vi "Main.vi"(7 "sweep rate, /min":dbl=0.2, 8 "sweep to:":dbl=-0.5, 9 "sweep":T6(radio)=enum."time_sweep") -> ()   [LabVIEW 2017] (continued)
                n297 = property on="Hyper Channel" class="DigNum (strict)"("Value"=w243) -> ()  [unwired: 2 in, 2 out]
              }
            }
          }
          frame #3 {
            # "Update current value of measured channel"
            n298 = property on="Monitor" class="Bool (strict)"() -> ("Value"=w279:bool)  [unwired: 2 in, 2 out]
            n299 = case shown="True" w279 {
              frame False {
              }
              frame True {
                n300 = stacked-sequence {
                  frame #0 {
                    # "Prepare the display format"
                    n301 = local read "2636A smua meas v"() -> (w285:bool)
                    n302 = local read "2636A smub meas v"() -> (w283:bool)
                    n303 = local read "2636A smub meas i"() -> (w282:bool)
                    n304 = local read "2636A smua meas i"() -> (w284:bool)
                    n305 = property on="sweep" class="RadioBtnsControl (strict)"() -> ("Value"=w280:T6)  [unwired: 2 in, 2 out]
                    n306 = Compound Arithmetic op=OR(w285, w284, w283, w282) -> (w281:bool)
                    n307 = case shown="True" w281 {
                      frame False {
                      }
                      frame True {
                        # "opens session for 2636a system sourcemeter"
                        n308 = local read "2336A addr"() -> (w334:refnum<visa-resource-name>)
                        n309 = VISA Close(VISA resource name=w334) -> ()  [unwired: 1 in, 1 out]
                      }
                    }
                    n310 = case shown="\"iTC\"" w280 {
                      frame "2400_1" {
                        # "add label for the first column in the datafile"
                        n311 = stacked-sequence {
                          frame #0 {
                            n312 = property on="data_caption" class="Str"("Value"="") -> ()  [unwired: 2 in, 2 out]
                            n313 = property on="Figure_axis" class="Arr (strict)"("Value"=string[] [] ("Figure_axis_string")) -> ()  [unwired: 2 in, 2 out]
                          }
                          frame #1 {
                            w288 = "V_sweep_2400_1" ("V_sweep")
                            n314 = Concatenate Strings(w288, "\t") -> (w290:string)
                            n315 = Build Array(w288) -> (w289:string[])
                            n316 = property on="data_caption" class="Str"("Value"=w290) -> ()  [unwired: 2 in, 2 out]
                            n317 = property on="Figure_axis" class="Arr (strict)"("Value"=w289) -> ()  [unwired: 2 in, 2 out]
                          }
                        }
                      }
                      frame "2400_2" {
                        n318 = stacked-sequence {
                          frame #0 {
                            n319 = property on="data_caption" class="Str"("Value"="") -> ()  [unwired: 2 in, 2 out]
                            n320 = property on="Figure_axis" class="Arr (strict)"("Value"=string[] [] ("Figure_axis_string")) -> ()  [unwired: 2 in, 2 out]
                          }
                          frame #1 {
                            w294 = "V_sweep_2400_2" ("V_sweep")
                            n321 = Build Array(w294) -> (w295:string[])
                            n322 = Concatenate Strings(w294, "\t") -> (w297:string)
                            n323 = property on="Figure_axis" class="Arr (strict)"("Value"=w295) -> ()  [unwired: 2 in, 2 out]
                            n324 = property on="data_caption" class="Str"("Value"=w297) -> ()  [unwired: 2 in, 2 out]
                          }
                        }
                      }
                      frame "2400_3" {
                        n325 = stacked-sequence {
                          frame #0 {
                            n326 = property on="data_caption" class="Str"("Value"="") -> ()  [unwired: 2 in, 2 out]
                            n327 = property on="Figure_axis" class="Arr (strict)"("Value"=string[] [] ("Figure_axis_string")) -> ()  [unwired: 2 in, 2 out]
                          }
                          frame #1 {
                            w300 = "V_sweep_2400_3" ("V_sweep")
                            n328 = Concatenate Strings(w300, "\t") -> (w303:string)
                            n329 = Build Array(w300) -> (w301:string[])
                            n330 = property on="data_caption" class="Str"("Value"=w303) -> ()  [unwired: 2 in, 2 out]
                            n331 = property on="Figure_axis" class="Arr (strict)"("Value"=w301) -> ()  [unwired: 2 in, 2 out]
                          }
                        }
                      }
                      frame "2636a_smua" {
                        n332 = stacked-sequence {
                          frame #0 {
                            n333 = property on="data_caption" class="Str"("Value"="") -> ()  [unwired: 2 in, 2 out]
                            n334 = property on="Figure_axis" class="Arr (strict)"("Value"=string[] [] ("Figure_axis_string")) -> ()  [unwired: 2 in, 2 out]
                          }
                          frame #1 {
                            w306 = "V_sweep_2636a_smua" ("V_sweep")
                            n335 = Concatenate Strings(w306, "\t") -> (w309:string)
                            n336 = Build Array(w306) -> (w307:string[])
                            n337 = property on="data_caption" class="Str"("Value"=w309) -> ()  [unwired: 2 in, 2 out]
                            n338 = property on="Figure_axis" class="Arr (strict)"("Value"=w307) -> ()  [unwired: 2 in, 2 out]
                          }
                        }
                      }
                      frame "2636a_smub" {
                        n339 = stacked-sequence {
                          frame #0 {
                            n340 = property on="data_caption" class="Str"("Value"="") -> ()  [unwired: 2 in, 2 out]
                            n341 = property on="Figure_axis" class="Arr (strict)"("Value"=string[] [] ("Figure_axis_string")) -> ()  [unwired: 2 in, 2 out]
                          }
                          frame #1 {
                            w312 = "V_sweep_2636a_smub" ("V_sweep")
                            n342 = Build Array(w312) -> (w313:string[])
                            n343 = Concatenate Strings(w312, "\t") -> (w315:string)
                            n344 = property on="Figure_axis" class="Arr (strict)"("Value"=w313) -> ()  [unwired: 2 in, 2 out]
                            n345 = property on="data_caption" class="Str"("Value"=w315) -> ()  [unwired: 2 in, 2 out]
                          }
                        }
                      }
                      frame "time_sweep", Default {
                        n346 = stacked-sequence {
                          frame #0 {
                            n347 = property on="data_caption" class="Str"("Value"="") -> ()  [unwired: 2 in, 2 out]
                            n348 = property on="Figure_axis" class="Arr (strict)"("Value"=string[] [] ("Figure_axis_string")) -> ()  [unwired: 2 in, 2 out]
                          }
                          frame #1 {
                            w318 = "time_sweep" ("V_sweep")
                            n349 = Build Array(w318) -> (w319:string[])
                            n350 = Concatenate Strings(w318, "\t") -> (w320:string)
                            n351 = property on="Figure_axis" class="Arr (strict)"("Value"=w319) -> ()  [unwired: 2 in, 2 out]
                            n352 = property on="data_caption" class="Str"("Value"=w320) -> ()  [unwired: 2 in, 2 out]
                          }
                        }
                      }
                      frame "iPS" {
                        # "sweep iPS"
                        n353 = stacked-sequence {
                          frame #0 {
                            n354 = property on="data_caption" class="Str"("Value"="") -> ()  [unwired: 2 in, 2 out]
                            n355 = property on="Figure_axis" class="Arr (strict)"("Value"=string[] [] ("Figure_axis_string")) -> ()  [unwired: 2 in, 2 out]
                          }
                          frame #1 {
                            w324 = "iPS_OutputField" ("V_sweep")
                            n356 = Build Array(w324) -> (w325:string[])
                            n357 = Concatenate Strings(w324, "\t") -> (w327:string)
                            n358 = property on="Figure_axis" class="Arr (strict)"("Value"=w325) -> ()  [unwired: 2 in, 2 out]
                            n359 = property on="data_caption" class="Str"("Value"=w327) -> ()  [unwired: 2 in, 2 out]
                          }
                        }
                      }
                      frame "iTC" {
                        n360 = stacked-sequence {
                          frame #0 {
                            n361 = property on="data_caption" class="Str"("Value"="") -> ()  [unwired: 2 in, 2 out]
                            n362 = property on="Figure_axis" class="Arr (strict)"("Value"=string[] ["", "SR830_1_ip", "SR830_1_oop", "SR830_2_ip", "SR830_2_oop", "2461_meas_v", "2461_meas_i", "2636A_smua_v", "2636A_smua_i", "formula"] ("Figure_axis")) -> ()  [unwired: 2 in, 2 out]
                          }
                          frame #1 {
                            w332 = "iTC_sample"
                            n363 = Build Array(w332) -> (w331:string[])
                            n364 = Concatenate Strings(w332, "\t") -> (w330:string)
                            n365 = property on="data_caption" class="Str"("Value"=w330) -> ()  [unwired: 2 in, 2 out]
                            n366 = property on="Figure_axis" class="Arr (strict)"("Value"=w331) -> ()  [unwired: 2 in, 2 out]
                          }
                        }
                      }
                    }
                  }
                  frame #1 {
                    # "this part constructs the first (text) line for the data file with names of all measured variables,\nalso constructs a text array contaning names of all measured variable for the \"ring\" (so parameter can be selected and plotted)"
                    n367 = stacked-sequence {
                      tunnel: [w335 _ _ _ _ _ _ _ _ _ _ _ _ _ _ _ _ _ _ _ _ _ _ _ _ _ _ _ _ _ _ _ _ _ _ _ _ _ _ _ _ _ _ _ _ _ _ _ _ _ _ _] -> _
                      frame #0 {
                        # "SR830 1 in phase (SR830_1_ip)"
                        n368 = local read "SR830 1 ip"() -> (w340:bool)
                        n369 = property on="Figure_axis" class="Arr (strict)"() -> ("Value"=w337:string[])  [unwired: 2 in, 2 out]
                        n370 = property on="data_caption" class="Str"() -> ("Value"=w339:string)  [unwired: 2 in, 2 out]
                        n371 = case shown="True" w340 {
                          tunnel: w339 -> [w342 w348]
                          tunnel: [w342 w347] -> w338
                          tunnel: w337 -> [w341 w345]
                          tunnel: [w341 w343] -> w336
                          frame False {
                            # "not measure SR830 1 in phase signal (SR830_1_ip)"
                          }
                          frame True {
                            w344 = "SR830_1_ip"
                            # "measure SR830 1 in phase signal (SR830_1_ip)"
                            n372 = local read "SR830 1 addr"() -> (w349:u8)
                            n373 = Number To Decimal String(number=w349) -> (decimal integer string=w350:string)  [unwired: 1 in]
                            n374 = GPIB Clear(3:w350) -> ()  [unwired: 1 in, 2 out]
                            n375 = Build Array (concatenate)(w345, w344) -> (w343:string[])
                            n376 = Concatenate Strings(w348, w344, "\t") -> (w347:string)
                          }
                        }
                        n377 = property on="Figure_axis" class="Arr (strict)"("Value"=w336) -> ()  [unwired: 2 in, 2 out]
                        n378 = property on="data_caption" class="Str"("Value"=w338) -> (error out=w335:errorcluster)  [unwired: 2 in, 1 out]
                      }
                      frame #1 {
                        # "SR830 1 out of phase (SR830_1_oop)"
                        n379 = local read "SR830 1 oop"() -> (w355:bool)
                        n380 = property on="Figure_axis" class="Arr (strict)"() -> ("Value"=w352:string[])  [unwired: 2 in, 2 out]
                        n381 = property on="data_caption" class="Str"() -> ("Value"=w354:string)  [unwired: 2 in, 2 out]
                        n382 = case shown="False" w355 {
                          tunnel: w354 -> [w357 w363]
                          tunnel: [w357 w362] -> w353
                          tunnel: w352 -> [w356 w360]
                          tunnel: [w356 w358] -> w351
                          frame False {
                            # "not measure SR830 1 out of phase signal (SR830_1_oop)"
                          }
                          frame True {
                            w359 = "SR830_1_oop"
                            # "measure SR830 1 out of phase signal (SR830_1_oop)"
                            n383 = local read "SR830 1 addr"() -> (w364:u8)
                            n384 = Number To Decimal String(number=w364) -> (decimal integer string=w365:string)  [unwired: 1 in]
                            n385 = GPIB Clear(3:w365) -> ()  [unwired: 1 in, 2 out]
                            n386 = Build Array (concatenate)(w360, w359) -> (w358:string[])
                            n387 = Concatenate Strings(w363, w359, "\t") -> (w362:string)
                          }
                        }
                        n388 = property on="Figure_axis" class="Arr (strict)"("Value"=w351) -> ()  [unwired: 2 in, 2 out]
                        n389 = property on="data_caption" class="Str"("Value"=w353) -> ()  [unwired: 2 in, 2 out]
                      }
                      frame #2 {
                        # "SR830 2 in phase (SR830_2_ip)"
                        n390 = local read "SR830 2 ip"() -> (w370:bool)
                        n391 = property on="Figure_axis" class="Arr (strict)"() -> ("Value"=w367:string[])  [unwired: 2 in, 2 out]
                        n392 = property on="data_caption" class="Str"() -> ("Value"=w369:string)  [unwired: 2 in, 2 out]
                        n393 = case shown="True" w370 {
                          tunnel: w369 -> [w372 w378]
                          tunnel: [w372 w377] -> w368
                          tunnel: w367 -> [w371 w375]
                          tunnel: [w371 w373] -> w366
                          frame False {
                            # "not measure SR830 2 in phase signal (SR830_2_ip)"
                          }
                          frame True {
                            w374 = "SR830_2_ip"
                            # "measure SR830 2 in phase signal (SR830_2_ip)"
                            n394 = local read "SR830 2 addr"() -> (w379:u8)
                            n395 = Number To Decimal String(number=w379) -> (decimal integer string=w380:string)  [unwired: 1 in]
                            n396 = GPIB Clear(3:w380) -> ()  [unwired: 1 in, 2 out]
                            n397 = Build Array (concatenate)(w375, w374) -> (w373:string[])
                            n398 = Concatenate Strings(w378, w374, "\t") -> (w377:string)
                          }
                        }
                        n399 = property on="Figure_axis" class="Arr (strict)"("Value"=w366) -> ()  [unwired: 2 in, 2 out]
                        n400 = property on="data_caption" class="Str"("Value"=w368) -> ()  [unwired: 2 in, 2 out]
                      }
                      frame #3 {
                        # "SR830 2 out of phase (SR830_2_oop)"
                        n401 = local read "SR830 2 oop"() -> (w385:bool)
                        n402 = property on="Figure_axis" class="Arr (strict)"() -> ("Value"=w382:string[])  [unwired: 2 in, 2 out]
                        n403 = property on="data_caption" class="Str"() -> ("Value"=w384:string)  [unwired: 2 in, 2 out]
                        n404 = case shown="False" w385 {
                          tunnel: w384 -> [w387 w393]
                          tunnel: [w387 w392] -> w383
                          tunnel: w382 -> [w386 w390]
                          tunnel: [w386 w388] -> w381
                          frame False {
                            # "not measure SR830 2 out of phase signal (SR830_2_oop)"
                          }
                          frame True {
                            w389 = "SR830_2_oop"
                            # "measure SR830 2 out of phase signal (SR830_2_oop)"
                            n405 = local read "SR830 2 addr"() -> (w394:u8)
                            n406 = Number To Decimal String(number=w394) -> (decimal integer string=w395:string)  [unwired: 1 in]
                            n407 = GPIB Clear(3:w395) -> ()  [unwired: 1 in, 2 out]
                            n408 = Build Array (concatenate)(w390, w389) -> (w388:string[])
                            n409 = Concatenate Strings(w393, w389, "\t") -> (w392:string)
                          }
                        }
                        n410 = property on="Figure_axis" class="Arr (strict)"("Value"=w381) -> ()  [unwired: 2 in, 2 out]
                        n411 = property on="data_caption" class="Str"("Value"=w383) -> ()  [unwired: 2 in, 2 out]
                      }
                      frame #4 {
                        # "SR830 3 in phase (SR830_3_ip)"
                        n412 = local read "SR830 3 ip"() -> (w400:bool)
                        n413 = property on="Figure_axis" class="Arr (strict)"() -> ("Value"=w397:string[])  [unwired: 2 in, 2 out]
                        n414 = property on="data_caption" class="Str"() -> ("Value"=w399:string)  [unwired: 2 in, 2 out]
                        n415 = case shown="True" w400 {
                          tunnel: w399 -> [w402 w408]
                          tunnel: [w402 w407] -> w398
                          tunnel: w397 -> [w401 w405]
                          tunnel: [w401 w403] -> w396
                          frame False {
                            # "not measure SR830 3 in phase signal (SR830_3_ip)"
                          }
                          frame True {
                            w404 = "SR830_3_ip"
                            # "measure SR830 3 in phase signal (SR830_3_ip)"
                            n416 = local read "SR830 3 addr"() -> (w409:u8)
                            n417 = Number To Decimal String(number=w409) -> (decimal integer string=w410:string)  [unwired: 1 in]
                            n418 = GPIB Clear(3:w410) -> ()  [unwired: 1 in, 2 out]
                            n419 = Build Array (concatenate)(w405, w404) -> (w403:string[])
                            n420 = Concatenate Strings(w408, w404, "\t") -> (w407:string)
                          }
                        }
                        n421 = property on="Figure_axis" class="Arr (strict)"("Value"=w396) -> ()  [unwired: 2 in, 2 out]
                        n422 = property on="data_caption" class="Str"("Value"=w398) -> ()  [unwired: 2 in, 2 out]
                      }
                      frame #5 {
                        # "SR830 3 out of phase (SR830_3_oop)"
                        n423 = local read "SR830 3 oop"() -> (w415:bool)
                        n424 = property on="Figure_axis" class="Arr (strict)"() -> ("Value"=w412:string[])  [unwired: 2 in, 2 out]
                        n425 = property on="data_caption" class="Str"() -> ("Value"=w414:string)  [unwired: 2 in, 2 out]
                        n426 = case shown="True" w415 {
                          tunnel: w414 -> [w417 w423]
                          tunnel: [w417 w422] -> w413
                          tunnel: w412 -> [w416 w420]
                          tunnel: [w416 w418] -> w411
                          frame False {
                            # "not measure SR830 3 out of phase signal (SR830_3_oop)"
                          }
                          frame True {
                            w419 = "SR830_3_oop"
                            # "measure SR830 3 out phase signal (SR830_3_oop)"
                            n427 = local read "SR830 3 addr"() -> (w424:u8)
                            n428 = Number To Decimal String(number=w424) -> (decimal integer string=w425:string)  [unwired: 1 in]
                            n429 = GPIB Clear(3:w425) -> ()  [unwired: 1 in, 2 out]
                            n430 = Build Array (concatenate)(w420, w419) -> (w418:string[])
                            n431 = Concatenate Strings(w423, w419, "\t") -> (w422:string)
                          }
                        }
                        n432 = property on="Figure_axis" class="Arr (strict)"("Value"=w411) -> ()  [unwired: 2 in, 2 out]
                        n433 = property on="data_caption" class="Str"("Value"=w413) -> ()  [unwired: 2 in, 2 out]
                      }
                      frame #6 {
                        # "SR830 4 in phase (SR830_4_ip)"
                        n434 = local read "SR830 4 ip"() -> (w430:bool)
                        n435 = property on="Figure_axis" class="Arr (strict)"() -> ("Value"=w427:string[])  [unwired: 2 in, 2 out]
                        n436 = property on="data_caption" class="Str"() -> ("Value"=w429:string)  [unwired: 2 in, 2 out]
                        n437 = case shown="False" w430 {
                          tunnel: w429 -> [w432 w438]
                          tunnel: [w432 w437] -> w428
                          tunnel: w427 -> [w431 w435]
                          tunnel: [w431 w433] -> w426
                          frame False {
                            # "not measure SR830 4 in phase signal (SR830_4_ip)"
                          }
                          frame True {
                            w434 = "SR830_4_ip"
                            # "measure SR830 4 in phase signal (SR830_4_ip)"
                            n438 = local read "SR830 4 addr"() -> (w439:u8)
                            n439 = Number To Decimal String(number=w439) -> (decimal integer string=w440:string)  [unwired: 1 in]
                            n440 = GPIB Clear(3:w440) -> ()  [unwired: 1 in, 2 out]
                            n441 = Build Array (concatenate)(w435, w434) -> (w433:string[])
                            n442 = Concatenate Strings(w438, w434, "\t") -> (w437:string)
                          }
                        }
                        n443 = property on="Figure_axis" class="Arr (strict)"("Value"=w426) -> ()  [unwired: 2 in, 2 out]
                        n444 = property on="data_caption" class="Str"("Value"=w428) -> ()  [unwired: 2 in, 2 out]
                      }
                      frame #7 {
                        # "SR830 4 out of phase (SR830_4_oop)"
                        n445 = local read "SR830 4 oop"() -> (w445:bool)
                        n446 = property on="Figure_axis" class="Arr (strict)"() -> ("Value"=w442:string[])  [unwired: 2 in, 2 out]
                        n447 = property on="data_caption" class="Str"() -> ("Value"=w444:string)  [unwired: 2 in, 2 out]
                        n448 = case shown="False" w445 {
                          tunnel: w444 -> [w447 w453]
                          tunnel: [w447 w452] -> w443
                          tunnel: w442 -> [w446 w450]
                          tunnel: [w446 w448] -> w441
                          frame False {
                            # "not measure SR830 4 out of phase signal (SR830_4_oop)"
                          }
                          frame True {
                            w449 = "SR830_4_oop"
                            # "measure SR830 4 out of phase signal (SR830_4_oop)"
                            n449 = local read "SR830 4 addr"() -> (w454:u8)
                            n450 = Number To Decimal String(number=w454) -> (decimal integer string=w455:string)  [unwired: 1 in]
                            n451 = GPIB Clear(3:w455) -> ()  [unwired: 1 in, 2 out]
                            n452 = Build Array (concatenate)(w450, w449) -> (w448:string[])
                            n453 = Concatenate Strings(w453, w449, "\t") -> (w452:string)
                          }
                        }
                        n454 = property on="Figure_axis" class="Arr (strict)"("Value"=w441) -> ()  [unwired: 2 in, 2 out]
                        n455 = property on="data_caption" class="Str"("Value"=w443) -> ()  [unwired: 2 in, 2 out]
                      }
                      frame #8 {
                        # "SR830 5 in phase (SR830_5_ip)"
                        n456 = local read "SR830 5 ip"() -> (w460:bool)
                        n457 = property on="Figure_axis" class="Arr (strict)"() -> ("Value"=w457:string[])  [unwired: 2 in, 2 out]
                        n458 = property on="data_caption" class="Str"() -> ("Value"=w459:string)  [unwired: 2 in, 2 out]
                        n459 = case shown="True" w460 {
                          tunnel: w459 -> [w462 w468]
                          tunnel: [w462 w467] -> w458
                          tunnel: w457 -> [w461 w465]
                          tunnel: [w461 w463] -> w456
                          frame False {
                            # "not measure SR830 5 in phase signal (SR830_5_ip)"
                          }
                          frame True {
                            w464 = "SR830_5_ip"
                            # "measure SR830 5 in phase signal (SR830_5_ip)"
                            n460 = local read "SR830 5 addr"() -> (w469:u8)
                            n461 = Number To Decimal String(number=w469) -> (decimal integer string=w470:string)  [unwired: 1 in]
                            n462 = GPIB Clear(3:w470) -> ()  [unwired: 1 in, 2 out]
                            n463 = Build Array (concatenate)(w465, w464) -> (w463:string[])
                            n464 = Concatenate Strings(w468, w464, "\t") -> (w467:string)
                          }
                        }
                        n465 = property on="Figure_axis" class="Arr (strict)"("Value"=w456) -> ()  [unwired: 2 in, 2 out]
                        n466 = property on="data_caption" class="Str"("Value"=w458) -> ()  [unwired: 2 in, 2 out]
                      }
                      frame #9 {
                        # "SR830 5 out of phase (SR830_5_oop)"
                        n467 = local read "SR830 5 oop"() -> (w475:bool)
                        n468 = property on="Figure_axis" class="Arr (strict)"() -> ("Value"=w472:string[])  [unwired: 2 in, 2 out]
                        n469 = property on="data_caption" class="Str"() -> ("Value"=w474:string)  [unwired: 2 in, 2 out]
                        n470 = case shown="True" w475 {
                          tunnel: w474 -> [w477 w483]
                          tunnel: [w477 w482] -> w473
                          tunnel: w472 -> [w476 w480]
                          tunnel: [w476 w478] -> w471
                          frame False {
                            # "not measure SR830 5 out of phase signal (SR830_5_oop)"
                          }
                          frame True {
                            w479 = "SR830_5_oop"
                            # "measure SR830 5 out of phase signal (SR830_5_oop)"
                            n471 = local read "SR830 5 addr"() -> (w484:u8)
                            n472 = Number To Decimal String(number=w484) -> (decimal integer string=w485:string)  [unwired: 1 in]
                            n473 = GPIB Clear(3:w485) -> ()  [unwired: 1 in, 2 out]
                            n474 = Build Array (concatenate)(w480, w479) -> (w478:string[])
                            n475 = Concatenate Strings(w483, w479, "\t") -> (w482:string)
                          }
                        }
                        n476 = property on="Figure_axis" class="Arr (strict)"("Value"=w471) -> ()  [unwired: 2 in, 2 out]
                        n477 = property on="data_caption" class="Str"("Value"=w473) -> ()  [unwired: 2 in, 2 out]
                      }
                      frame #10 {
                        # "SR830 6 in phase (SR830_6_ip)"
                        n478 = property on="SR830_6_ip" class="Bool (strict)"() -> ("Value"=w486:bool)  [unwired: 2 in, 2 out]
                        n479 = property on="Figure_axis" class="Arr (strict)"() -> ("Value"=w488:string[])  [unwired: 2 in, 2 out]
                        n480 = property on="data_caption" class="Str"() -> ("Value"=w490:string)  [unwired: 2 in, 2 out]
                        n481 = case shown="True" w486 {
                          tunnel: w490 -> [w492 w498]
                          tunnel: [w492 w497] -> w489
                          tunnel: w488 -> [w491 w495]
                          tunnel: [w491 w493] -> w487
                          frame False {
                            # "not measure SR830 6 in phase signal (SR830_6_ip)"
                          }
                          frame True {
                            w494 = "SR830_6_ip"
                            # "measure SR830 6 in phase signal (SR830_6_ip)"
                            n482 = local read "SR830_6"() -> (w499:u8)
                            n483 = Number To Decimal String(number=w499) -> (decimal integer string=w500:string)  [unwired: 1 in]
                            n484 = GPIB Clear(3:w500) -> ()  [unwired: 1 in, 2 out]
                            n485 = Build Array (concatenate)(w495, w494) -> (w493:string[])
                            n486 = Concatenate Strings(w498, w494, "\t") -> (w497:string)
                          }
                        }
                        n487 = property on="Figure_axis" class="Arr (strict)"("Value"=w487) -> ()  [unwired: 2 in, 2 out]
                        n488 = property on="data_caption" class="Str"("Value"=w489) -> ()  [unwired: 2 in, 2 out]
                      }
                      frame #11 {
                        # "SR830 6 out of phase (SR830_6_oop)"
                        n489 = local read "SR830_6_oop"() -> (w505:bool)
                        n490 = property on="Figure_axis" class="Arr (strict)"() -> ("Value"=w502:string[])  [unwired: 2 in, 2 out]
                        n491 = property on="data_caption" class="Str"() -> ("Value"=w504:string)  [unwired: 2 in, 2 out]
                        n492 = case shown="False" w505 {
                          tunnel: w504 -> [w507 w513]
                          tunnel: [w507 w512] -> w503
                          tunnel: w502 -> [w506 w510]
                          tunnel: [w506 w508] -> w501
                          frame False {
                            # "not measure SR830 6 out of phase signal (SR830_6_oop)"
                          }
                          frame True {
                            w509 = "SR830_6_oop"
                            # "measure SR830 6 out of phase signal (SR830_6_oop)"
                            n493 = local read "SR830_6"() -> (w514:u8)
                            n494 = Number To Decimal String(number=w514) -> (decimal integer string=w515:string)  [unwired: 1 in]
                            n495 = GPIB Clear(3:w515) -> ()  [unwired: 1 in, 2 out]
                            n496 = Build Array (concatenate)(w510, w509) -> (w508:string[])
                            n497 = Concatenate Strings(w513, w509, "\t") -> (w512:string)
                          }
                        }
                        n498 = property on="Figure_axis" class="Arr (strict)"("Value"=w501) -> ()  [unwired: 2 in, 2 out]
                        n499 = property on="data_caption" class="Str"("Value"=w503) -> ()  [unwired: 2 in, 2 out]
                      }
                      frame #12 {
                        # "SR830 7 in phase (SR830_7_ip)"
                        n500 = local read "SR830_7_ip"() -> (w516:bool)
                        n501 = property on="Figure_axis" class="Arr (strict)"() -> ("Value"=w518:string[])  [unwired: 2 in, 2 out]
                        n502 = property on="data_caption" class="Str"() -> ("Value"=w520:string)  [unwired: 2 in, 2 out]
                        n503 = case shown="True" w516 {
                          tunnel: w520 -> [w522 w528]
                          tunnel: [w522 w527] -> w519
                          tunnel: w518 -> [w521 w525]
                          tunnel: [w521 w523] -> w517
                          frame False {
                            # "not measure SR830 7 in phase signal (SR830_7_ip)"
                          }
                          frame True {
                            w524 = "SR830_7_ip"
                            # "measure SR830 7 in phase signal (SR830_7_ip)"
                            n504 = local read "SR830_7"() -> (w529:u8)
                            n505 = Number To Decimal String(number=w529) -> (decimal integer string=w530:string)  [unwired: 1 in]
                            n506 = GPIB Clear(3:w530) -> ()  [unwired: 1 in, 2 out]
                            n507 = Build Array (concatenate)(w525, w524) -> (w523:string[])
                            n508 = Concatenate Strings(w528, w524, "\t") -> (w527:string)
                          }
                        }
                        n509 = property on="Figure_axis" class="Arr (strict)"("Value"=w517) -> ()  [unwired: 2 in, 2 out]
                        n510 = property on="data_caption" class="Str"("Value"=w519) -> ()  [unwired: 2 in, 2 out]
                      }
                      frame #13 {
                        # "SR830 7 out of phase (SR830_7_oop)"
                        n511 = local read "SR830_7_oop"() -> (w535:bool)
                        n512 = property on="Figure_axis" class="Arr (strict)"() -> ("Value"=w532:string[])  [unwired: 2 in, 2 out]
                        n513 = property on="data_caption" class="Str"() -> ("Value"=w534:string)  [unwired: 2 in, 2 out]
                        n514 = case shown="True" w535 {
                          tunnel: w534 -> [w537 w543]
                          tunnel: [w537 w542] -> w533
                          tunnel: w532 -> [w536 w540]
                          tunnel: [w536 w538] -> w531
                          frame False {
                            # "not measure SR830 7 out of phase signal (SR830_7_oop)"
                          }
                          frame True {
                            w539 = "SR830_7_oop"
                            # "measure SR830 7 out of phase signal (SR830_7_oop)"
                            n515 = local read "SR830_7"() -> (w544:u8)
                            n516 = Number To Decimal String(number=w544) -> (decimal integer string=w545:string)  [unwired: 1 in]
                            n517 = GPIB Clear(3:w545) -> ()  [unwired: 1 in, 2 out]
                            n518 = Build Array (concatenate)(w540, w539) -> (w538:string[])
                            n519 = Concatenate Strings(w543, w539, "\t") -> (w542:string)
                          }
                        }
                        n520 = property on="Figure_axis" class="Arr (strict)"("Value"=w531) -> ()  [unwired: 2 in, 2 out]
                        n521 = property on="data_caption" class="Str"("Value"=w533) -> ()  [unwired: 2 in, 2 out]
                      }
                      frame #14 {
                        # "SR830 8 in phase (SR830_8_ip)"
                        n522 = local read "SR830_8_ip"() -> (w546:bool)
                        n523 = property on="Figure_axis" class="Arr (strict)"() -> ("Value"=w548:string[])  [unwired: 2 in, 2 out]
                        n524 = property on="data_caption" class="Str"() -> ("Value"=w550:string)  [unwired: 2 in, 2 out]
                        n525 = case shown="True" w546 {
                          tunnel: w550 -> [w552 w558]
                          tunnel: [w552 w557] -> w549
                          tunnel: w548 -> [w551 w555]
                          tunnel: [w551 w553] -> w547
                          frame False {
                            # "not measure SR830 8 in phase signal (SR830_8_ip)"
                          }
                          frame True {
                            w554 = "SR830_8_ip"
                            # "measure SR830 8 in phase signal (SR830_8_ip)"
                            n526 = local read "SR830_8"() -> (w559:u8)
                            n527 = Number To Decimal String(number=w559) -> (decimal integer string=w560:string)  [unwired: 1 in]
                            n528 = GPIB Clear(3:w560) -> ()  [unwired: 1 in, 2 out]
                            n529 = Build Array (concatenate)(w555, w554) -> (w553:string[])
                            n530 = Concatenate Strings(w558, w554, "\t") -> (w557:string)
                          }
                        }
                        n531 = property on="Figure_axis" class="Arr (strict)"("Value"=w547) -> ()  [unwired: 2 in, 2 out]
                        n532 = property on="data_caption" class="Str"("Value"=w549) -> ()  [unwired: 2 in, 2 out]
                      }
                      frame #15 {
                        # "SR830 8 out phase (SR830_8_oop)"
                        n533 = local read "SR830_8_oop"() -> (w561:bool)
                        n534 = property on="Figure_axis" class="Arr (strict)"() -> ("Value"=w563:string[])  [unwired: 2 in, 2 out]
                        n535 = property on="data_caption" class="Str"() -> ("Value"=w565:string)  [unwired: 2 in, 2 out]
                        n536 = case shown="True" w561 {
                          tunnel: w565 -> [w567 w573]
                          tunnel: [w567 w572] -> w564
                          tunnel: w563 -> [w566 w570]
                          tunnel: [w566 w568] -> w562
                          frame False {
                            # "not measure SR830 8 out phase signal (SR830_8_oop)"
                          }
                          frame True {
                            w569 = "SR830_8_oop"
                            # "measure SR830 8 out phase signal (SR830_8_00p)"
                            n537 = local read "SR830_8"() -> (w574:u8)
                            n538 = Number To Decimal String(number=w574) -> (decimal integer string=w575:string)  [unwired: 1 in]
                            n539 = GPIB Clear(3:w575) -> ()  [unwired: 1 in, 2 out]
                            n540 = Build Array (concatenate)(w570, w569) -> (w568:string[])
                            n541 = Concatenate Strings(w573, w569, "\t") -> (w572:string)
                          }
                        }
                        n542 = property on="Figure_axis" class="Arr (strict)"("Value"=w562) -> ()  [unwired: 2 in, 2 out]
                        n543 = property on="data_caption" class="Str"("Value"=w564) -> ()  [unwired: 2 in, 2 out]
                      }
                      frame #16 {
                        # "MFLI_V1"
                        n544 = property on="MFLI_1" class="Str" props=["Value"]() -> ()  [unwired: 2 in, 3 out]
                        n545 = property on="MFLI_V1" class="Bool (strict)"() -> ("Value"=w576:bool)  [unwired: 2 in, 2 out]
                        n546 = property on="data_caption" class="Str"() -> ("Value"=w580:string)  [unwired: 2 in, 2 out]
                        n547 = property on="Figure_axis" class="Arr (strict)"() -> ("Value"=w578:string[])  [unwired: 2 in, 2 out]
                        n548 = case shown="True" w576 {
                          tunnel: w580 -> [w582 w592]
                          tunnel: [w582 w591] -> w579
                          tunnel: w578 -> [w581 w590]
                          tunnel: [w581 w589] -> w577
                          frame False {
                            # "not measure 2461 voltage (2461_meas_v)"
                          }
                          frame True {
                            w587 = "MFLI_Vy_1"
                            w588 = "MFLI_Vx_1"
                            w586 = "\t"
                            w585 = "MFLI_freq_1"
                            n549 = property on="HandleOut" class="Clust (strict)"() -> ("Value"=w584:T5)  [unwired: 2 in, 2 out]
                            n550 = Unbundle(w584) -> ("Connected"=w583:bool)  [unwired: 5 out]
                            n551 = case shown="False" w583 {
                              frame False {
                                n552 = property on="MFLI_1" class="Str"() -> ("Value"=w595:string)  [unwired: 2 in, 2 out]
                                n553 = call <instrlib>:"ziOpen.vi"("Address"=w595) -> ("HandleOut"=w594:T5)  [unwired: 3 in, 2 out]
                                n554 = call <instrlib>:"ziCheckVersion.vi"("Handle In"=w594) -> ("Handle Out"=w593:T5)  [unwired: 12 in, 2 out]
                                n555 = property on="HandleOut" class="Clust (strict)"("Value"=w593) -> ()  [unwired: 2 in, 2 out]
                              }
                              frame True {
                              }
                            }
                            n556 = Build Array (concatenate)(w590, w588, w587, w585) -> (w589:string[])
                            n557 = Concatenate Strings(w592, w588, w586, w587, w586, w585, w586) -> (w591:string)
                          }
                        }
                        n558 = property on="Figure_axis" class="Arr (strict)"("Value"=w577) -> ()  [unwired: 2 in, 2 out]
                        n559 = property on="data_caption" class="Str"("Value"=w579) -> ()  [unwired: 2 in, 2 out]
                      }
                      frame #17 {
                        # "MFLI_I1"
                        n560 = property on="MFLI_I1" class="Bool (strict)"() -> ("Value"=w596:bool)  [unwired: 2 in, 2 out]
                        n561 = property on="data_caption" class="Str"() -> ("Value"=w600:string)  [unwired: 2 in, 2 out]
                        n562 = property on="Figure_axis" class="Arr (strict)"() -> ("Value"=w598:string[])  [unwired: 2 in, 2 out]
                        n563 = case shown="True" w596 {
                          tunnel: w600 -> [w602 w612]
                          tunnel: [w602 w611] -> w599
                          tunnel: w598 -> [w601 w610]
                          tunnel: [w601 w609] -> w597
                          frame False {
                            # "not measure 2461 voltage (2461_meas_v)"
                          }
                          frame True {
                            w607 = "MFLI_Iy-1"
                            w608 = "MFLI_Ix_1"
                            w606 = "\t"
                            w605 = "MFLI_freq_1"
                            n564 = property on="HandleOut" class="Clust (strict)"() -> ("Value"=w604:T5)  [unwired: 2 in, 2 out]
                            n565 = Unbundle(w604) -> ("Connected"=w603:bool)  [unwired: 5 out]
                            n566 = case shown="False" w603 {
                              frame False {
                                n567 = property on="MFLI_1" class="Str"() -> ("Value"=w615:string)  [unwired: 2 in, 2 out]
                                n568 = call <instrlib>:"ziOpen.vi"("Address"=w615) -> ("HandleOut"=w614:T5)  [unwired: 3 in, 2 out]
                                n569 = call <instrlib>:"ziCheckVersion.vi"("Handle In"=w614) -> ("Handle Out"=w613:T5)  [unwired: 12 in, 2 out]
                                n570 = property on="HandleOut" class="Clust (strict)"("Value"=w613) -> ()  [unwired: 2 in, 2 out]
                              }
                              frame True {
                              }
                            }
                            n571 = Build Array (concatenate)(w610, w608, w607, w605) -> (w609:string[])
                            n572 = Concatenate Strings(w612, w608, w606, w607, w606, w605, w606) -> (w611:string)
                          }
                        }
                        n573 = property on="Figure_axis" class="Arr (strict)"("Value"=w597) -> ()  [unwired: 2 in, 2 out]
                        n574 = property on="data_caption" class="Str"("Value"=w599) -> ()  [unwired: 2 in, 2 out]
                      }
                      frame #18 {
                        # "MFLI_V 2"
                        n575 = local read "MFLI_V2"() -> (w616:bool)
                        n576 = property on="data_caption" class="Str"() -> ("Value"=w620:string)  [unwired: 2 in, 2 out]
                        n577 = property on="Figure_axis" class="Arr (strict)"() -> ("Value"=w618:string[])  [unwired: 2 in, 2 out]
                        n578 = case shown="True" w616 {
                          tunnel: w620 -> [w622 w632]
                          tunnel: [w622 w631] -> w619
                          tunnel: w618 -> [w621 w630]
                          tunnel: [w621 w629] -> w617
                          frame False {
                          }
                          frame True {
                            w627 = "MFLI_Vy_2"
                            w628 = "MFLI_Vx_2"
                            w626 = "\t"
                            w625 = "MFLI_freq_2"
                            n579 = property on="Handle Out 2" class="Clust (strict)"() -> ("Value"=w624:T5)  [unwired: 2 in, 2 out]
                            n580 = Unbundle(w624) -> ("Connected"=w623:bool)  [unwired: 5 out]
                            n581 = case shown="False" w623 {
                              frame False {
                                n582 = local read "MFLI_2"() -> (w633:string)
                                n583 = call <instrlib>:"ziOpen.vi"("Address"=w633) -> ("HandleOut"=w635:T5)  [unwired: 3 in, 2 out]
                                n584 = call <instrlib>:"ziCheckVersion.vi"("Handle In"=w635) -> ("Handle Out"=w634:T5)  [unwired: 12 in, 2 out]
                                n585 = property on="Handle Out 2" class="Clust (strict)"("Value"=w634) -> ()  [unwired: 2 in, 2 out]
                              }
                              frame True {
                              }
                            }
                            n586 = Build Array (concatenate)(w630, w628, w627, w625) -> (w629:string[])
                            n587 = Concatenate Strings(w632, w628, w626, w627, w626, w625, w626) -> (w631:string)
                          }
                        }
                        n588 = property on="Figure_axis" class="Arr (strict)"("Value"=w617) -> ()  [unwired: 2 in, 2 out]
                        n589 = property on="data_caption" class="Str"("Value"=w619) -> ()  [unwired: 2 in, 2 out]
                      }
                      frame #19 {
                        # "MFLI_I 2"
                        n590 = local read "MFLI_I2"() -> (w636:bool)
                        n591 = property on="data_caption" class="Str"() -> ("Value"=w640:string)  [unwired: 2 in, 2 out]
                        n592 = property on="Figure_axis" class="Arr (strict)"() -> ("Value"=w638:string[])  [unwired: 2 in, 2 out]
                        n593 = case shown="True" w636 {
                          tunnel: w640 -> [w642 w652]
                          tunnel: [w642 w651] -> w639
                          tunnel: w638 -> [w641 w650]
                          tunnel: [w641 w649] -> w637
                          frame False {
                            # "not measure 2461 voltage (2461_meas_v)"
                          }
                          frame True {
                            w647 = "MFLI_Iy_2"
                            w648 = "MFLI_Ix_2"
                            w646 = "\t"
                            w645 = "MFLI_freq_2"
                            n594 = property on="Handle Out 2" class="Clust (strict)"() -> ("Value"=w644:T5)  [unwired: 2 in, 2 out]
                            n595 = Unbundle(w644) -> ("Connected"=w643:bool)  [unwired: 5 out]
                            n596 = case shown="False" w643 {
                              frame False {
                                n597 = local read "MFLI_2"() -> (w653:string)
                                n598 = call <instrlib>:"ziOpen.vi"("Address"=w653) -> ("HandleOut"=w655:T5)  [unwired: 3 in, 2 out]
                                n599 = call <instrlib>:"ziCheckVersion.vi"("Handle In"=w655) -> ("Handle Out"=w654:T5)  [unwired: 12 in, 2 out]
                                n600 = property on="Handle Out 2" class="Clust (strict)"("Value"=w654) -> ()  [unwired: 2 in, 2 out]
                              }
                              frame True {
                              }
                            }
                            n601 = Build Array (concatenate)(w650, w648, w647, w645) -> (w649:string[])
                            n602 = Concatenate Strings(w652, w648, w646, w647, w646, w645, w646) -> (w651:string)
                          }
                        }
                        n603 = property on="Figure_axis" class="Arr (strict)"("Value"=w637) -> ()  [unwired: 2 in, 2 out]
                        n604 = property on="data_caption" class="Str"("Value"=w639) -> ()  [unwired: 2 in, 2 out]
                      }
                      frame #20 {
                        # "2400 1 voltage measure (2400_1_v)"
                        n605 = local read "2400 1 meas v"() -> (w660:bool)
                        n606 = property on="Figure_axis" class="Arr (strict)"() -> ("Value"=w657:string[])  [unwired: 2 in, 2 out]
                        n607 = property on="data_caption" class="Str"() -> ("Value"=w659:string)  [unwired: 2 in, 2 out]
                        n608 = case shown="False" w660 {
                          tunnel: w659 -> [w662 w668]
                          tunnel: [w662 w667] -> w658
                          tunnel: w657 -> [w661 w665]
                          tunnel: [w661 w663] -> w656
                          frame False {
                            # "not measure 2400 1 voltage (2400_1_v)"
                          }
                          frame True {
                            w664 = "2400_1_v"
                            # "measure 2400 1 voltage (2400_1_v)"
                            n609 = local read "2400 1 addr"() -> (w669:u8)
                            n610 = Number To Decimal String(number=w669) -> (decimal integer string=w670:string)  [unwired: 1 in]
                            n611 = GPIB Clear(3:w670) -> ()  [unwired: 1 in, 2 out]
                            n612 = Build Array (concatenate)(w665, w664) -> (w663:string[])
                            n613 = Concatenate Strings(w668, w664, "\t") -> (w667:string)
                          }
                        }
                        n614 = property on="Figure_axis" class="Arr (strict)"("Value"=w656) -> ()  [unwired: 2 in, 2 out]
                        n615 = property on="data_caption" class="Str"("Value"=w658) -> ()  [unwired: 2 in, 2 out]
                      }
                      frame #21 {
                        # "2400 1 current measure (2400_1_i)"
                        n616 = local read "2400 1 meas i"() -> (w675:bool)
                        n617 = property on="Figure_axis" class="Arr (strict)"() -> ("Value"=w672:string[])  [unwired: 2 in, 2 out]
                        n618 = property on="data_caption" class="Str"() -> ("Value"=w674:string)  [unwired: 2 in, 2 out]
                        n619 = case shown="False" w675 {
                          tunnel: w674 -> [w677 w683]
                          tunnel: [w677 w682] -> w673
                          tunnel: w672 -> [w676 w680]
                          tunnel: [w676 w678] -> w671
                          frame False {
                            # "not measure 2400 1 current (2400_1_i)"
                          }
                          frame True {
                            w679 = "2400_1_i"
                            # "measure 2400 1 current (2400_1_i)"
                            n620 = local read "2400 1 addr"() -> (w684:u8)
                            n621 = Number To Decimal String(number=w684) -> (decimal integer string=w685:string)  [unwired: 1 in]
                            n622 = GPIB Clear(3:w685) -> ()  [unwired: 1 in, 2 out]
                            n623 = Build Array (concatenate)(w680, w679) -> (w678:string[])
                            n624 = Concatenate Strings(w683, w679, "\t") -> (w682:string)
                          }
                        }
                        n625 = property on="Figure_axis" class="Arr (strict)"("Value"=w671) -> ()  [unwired: 2 in, 2 out]
                        n626 = property on="data_caption" class="Str"("Value"=w673) -> ()  [unwired: 2 in, 2 out]
                      }
                      frame #22 {
                        # "2400 2 voltage measure (2400_2_v)"
                        n627 = local read "2400 2 meas v"() -> (w690:bool)
                        n628 = property on="Figure_axis" class="Arr (strict)"() -> ("Value"=w687:string[])  [unwired: 2 in, 2 out]
                        n629 = property on="data_caption" class="Str"() -> ("Value"=w689:string)  [unwired: 2 in, 2 out]
                        n630 = case shown="False" w690 {
                          tunnel: w689 -> [w692 w698]
                          tunnel: [w692 w697] -> w688
                          tunnel: w687 -> [w691 w695]
                          tunnel: [w691 w693] -> w686
                          frame False {
                            # "not measure 2400 2 voltage (2400_2_v)"
                          }
                          frame True {
                            w694 = "2400_2_v"
                            # "measure 2400 2 voltage (2400_2_v)"
                            n631 = local read "2400 2 addr"() -> (w699:u8)
                            n632 = Number To Decimal String(number=w699) -> (decimal integer string=w700:string)  [unwired: 1 in]
                            n633 = GPIB Clear(3:w700) -> ()  [unwired: 1 in, 2 out]
                            n634 = Build Array (concatenate)(w695, w694) -> (w693:string[])
                            n635 = Concatenate Strings(w698, w694, "\t") -> (w697:string)
                          }
                        }
                        n636 = property on="Figure_axis" class="Arr (strict)"("Value"=w686) -> ()  [unwired: 2 in, 2 out]
                        n637 = property on="data_caption" class="Str"("Value"=w688) -> ()  [unwired: 2 in, 2 out]
                      }
                      frame #23 {
                        # "2400 2 current measure (2400_2_i)"
                        n638 = local read "2400 2 meas i"() -> (w705:bool)
                        n639 = property on="Figure_axis" class="Arr (strict)"() -> ("Value"=w702:string[])  [unwired: 2 in, 2 out]
                        n640 = property on="data_caption" class="Str"() -> ("Value"=w704:string)  [unwired: 2 in, 2 out]
                        n641 = case shown="False" w705 {
                          tunnel: w704 -> [w707 w713]
                          tunnel: [w707 w712] -> w703
                          tunnel: w702 -> [w706 w710]
                          tunnel: [w706 w708] -> w701
                          frame False {
                            # "not measure 2400 2 current (2400_2_i)"
                          }
                          frame True {
                            w709 = "2400_2_i"
                            # "measure 2400 2 current (2400_2_i)"
                            n642 = local read "2400 2 addr"() -> (w714:u8)
                            n643 = Number To Decimal String(number=w714) -> (decimal integer string=w715:string)  [unwired: 1 in]
                            n644 = GPIB Clear(3:w715) -> ()  [unwired: 1 in, 2 out]
                            n645 = Build Array (concatenate)(w710, w709) -> (w708:string[])
                            n646 = Concatenate Strings(w713, w709, "\t") -> (w712:string)
                          }
                        }
                        n647 = property on="Figure_axis" class="Arr (strict)"("Value"=w701) -> ()  [unwired: 2 in, 2 out]
                        n648 = property on="data_caption" class="Str"("Value"=w703) -> ()  [unwired: 2 in, 2 out]
                      }
                      frame #24 {
                        # "2400 3 voltage measure (2400_3_v)"
                        n649 = local read "2400 3 meas v"() -> (w720:bool)
                        n650 = property on="Figure_axis" class="Arr (strict)"() -> ("Value"=w717:string[])  [unwired: 2 in, 2 out]
                        n651 = property on="data_caption" class="Str"() -> ("Value"=w719:string)  [unwired: 2 in, 2 out]
                        n652 = case shown="False" w720 {
                          tunnel: w719 -> [w722 w728]
                          tunnel: [w722 w727] -> w718
                          tunnel: w717 -> [w721 w725]
                          tunnel: [w721 w723] -> w716
                          frame False {
                            # "not measure 2400 3 voltage (2400_3_v)"
                          }
                          frame True {
                            w724 = "2400_3_v"
                            # "measure 2400 3 voltage (2400_3_v)"
                            n653 = local read "2400 3 addr"() -> (w729:u8)
                            n654 = Number To Decimal String(number=w729) -> (decimal integer string=w730:string)  [unwired: 1 in]
                            n655 = GPIB Clear(3:w730) -> ()  [unwired: 1 in, 2 out]
                            n656 = Build Array (concatenate)(w725, w724) -> (w723:string[])
                            n657 = Concatenate Strings(w728, w724, "\t") -> (w727:string)
                          }
                        }
                        n658 = property on="Figure_axis" class="Arr (strict)"("Value"=w716) -> ()  [unwired: 2 in, 2 out]
                        n659 = property on="data_caption" class="Str"("Value"=w718) -> ()  [unwired: 2 in, 2 out]
                      }
                      frame #25 {
                        # "2400 3 current measure (2400_3_i)"
                        n660 = local read "2400 3 meas i"() -> (w735:bool)
                        n661 = property on="Figure_axis" class="Arr (strict)"() -> ("Value"=w732:string[])  [unwired: 2 in, 2 out]
                        n662 = property on="data_caption" class="Str"() -> ("Value"=w734:string)  [unwired: 2 in, 2 out]
                        n663 = case shown="True" w735 {
                          tunnel: w734 -> [w737 w743]
                          tunnel: [w737 w742] -> w733
                          tunnel: w732 -> [w736 w740]
                          tunnel: [w736 w738] -> w731
                          frame False {
                            # "not measure 2400 3 current (2400_3_i)"
                          }
                          frame True {
                            w739 = "2400_3_i"
                            # "measure 2400 3 current (2400_3_i)"
                            n664 = local read "2400 3 addr"() -> (w744:u8)
                            n665 = Number To Decimal String(number=w744) -> (decimal integer string=w745:string)  [unwired: 1 in]
                            n666 = GPIB Clear(3:w745) -> ()  [unwired: 1 in, 2 out]
                            n667 = Build Array (concatenate)(w740, w739) -> (w738:string[])
                            n668 = Concatenate Strings(w743, w739, "\t") -> (w742:string)
                          }
                        }
                        n669 = property on="Figure_axis" class="Arr (strict)"("Value"=w731) -> ()  [unwired: 2 in, 2 out]
                        n670 = property on="data_caption" class="Str"("Value"=w733) -> ()  [unwired: 2 in, 2 out]
                      }
                      frame #26 {
                        # "2182A 1 channel 1 measure (2182A_1_ch1)"
                        n671 = local read "2182A 1 ch1"() -> (w750:bool)
                        n672 = property on="Figure_axis" class="Arr (strict)"() -> ("Value"=w747:string[])  [unwired: 2 in, 2 out]
                        n673 = property on="data_caption" class="Str"() -> ("Value"=w749:string)  [unwired: 2 in, 2 out]
                        n674 = case shown="False" w750 {
